vi "mtrADCtoAmps(SubVI).vi"(11 "ADCcurrent":dbl) -> (3 "Numeric":dbl)   [LabVIEW 2013]
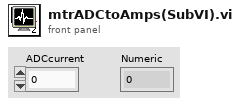
[diagram p1: front panel]
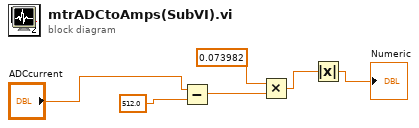
[diagram p0: block diagram]
diagram:
  n1 = Subtract(x="ADCcurrent", y=512.0) -> (x-y=w4:dbl)
  n2 = Multiply(x=0.073982, y=w4) -> (x*y=w1:dbl)
  n3 = Absolute Value(x=w1) -> (abs(x)=→"Numeric":dbl)
